vi "MFC Profile Generator.vi"(9 "Staircase Parameters":T1={"Step Time Duration"=1, "Step Flow Rate"=0.0, "Steps"=1, "Valve Open Start"=1, "Recovery"=FALSE, "Repeats"=1} {"Repeats" min=1 max=1000 step=1; "Valve Open Start" min=1 max=1000 step=1; "Steps" min=1 max=1000 step=1; "Step Flow Rate" min=0.0 max=200.0 scale=0.0..200.0; "Step Time Duration" min=1 max=1000 step=1}, 10 "Heaviside Step Parameters":T3 {"Valve Open Start" min=1 max=1000 step=1; "Valve Open Repeats" min=1 max=1000 step=1; "MFC Flow Rate" min=0.0 max=200.0 scale=0.0..200.0; "Valve Open Duration" min=1 max=1000 step=1}, 11 "Challenge Profile Type":T2) -> (3 "MFC Challenge Profile":dbl[](graph))   [LabVIEW 2011]
uses:
  Controls/MFC Challenge Profile - Heaviside Step.ctl
  Controls/MFC Challen Profile Type.ctl
  Controls/MFC Challenge Profile - Staircase.ctl
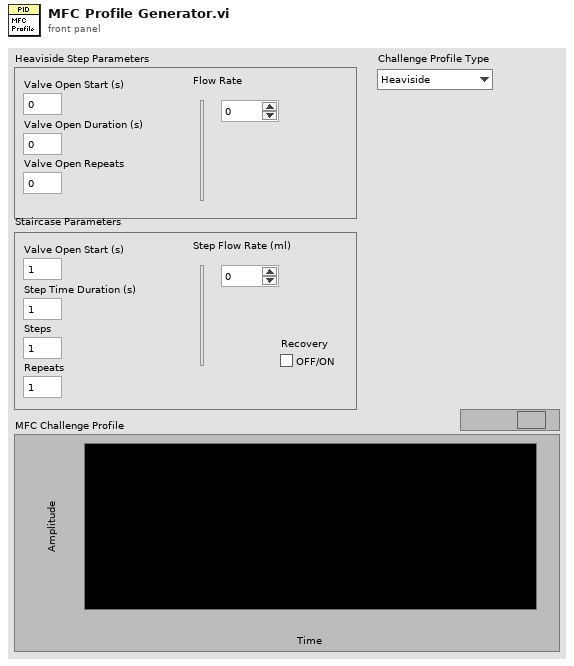
[diagram p1: front panel]
types:
  T1 = typedef "MFC Challenge Profile - Staircase.ctl" = cluster{"Step Time Duration":u16, "Step Flow Rate":dbl, "Steps":u16, "Valve Open Start":u16, "Recovery":bool, "Repeats":u16}
  T2 = typedef "MFC Challen Profile Type.ctl" = enum16{"Heaviside", "Staircase"}
  T3 = typedef "MFC Challenge Profile - Heaviside Step.ctl" = cluster{"Valve Open Duration":u16, "MFC Flow Rate":dbl, "Valve Open Repeats":u16, "Valve Open Start":u16}
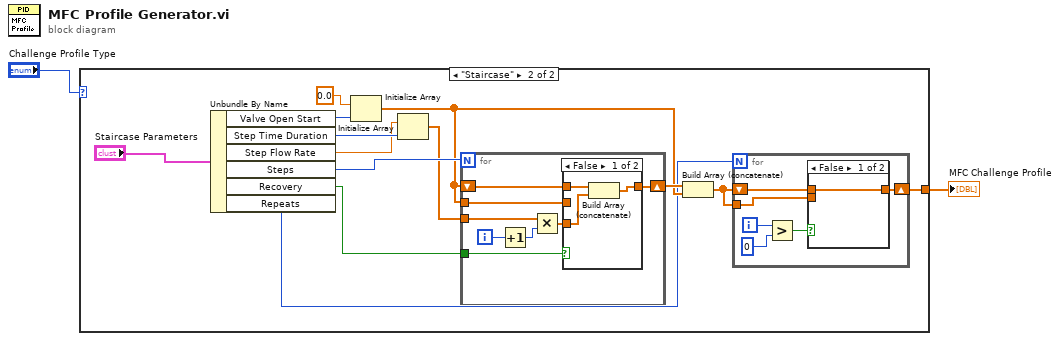
[diagram p0: block diagram]
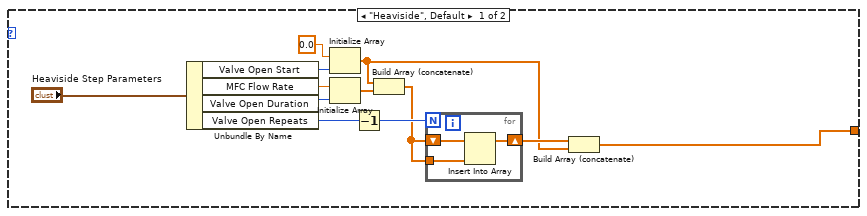
[diagram p2: hidden frame]
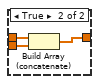
[diagram p3: hidden frame]
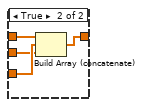
[diagram p4: hidden frame]
diagram:
  n1 = case shown="\"Staircase\"" "Challenge Profile Type" {
    tunnel: [w3 w18] -> w1
    frame "Heaviside", Default {
      n2 = Unbundle By Name("Heaviside Step Parameters") -> ("Valve Open Start"=w7:u16, "MFC Flow Rate"=w9:dbl, "Valve Open Duration"=w10:u16, "Valve Open Repeats"=w13:u16)
      n3 = Initialize Array(0.0 ("element"), w7) -> (w4:dbl[])
      n4 = Initialize Array(w9, w10) -> (w11:dbl[])
      n5 = Decrement(x=w13) -> (x-1=w14:u16)
      n6 = Build Array (concatenate)(w4, w11) -> (w12:dbl[])
      n7 = for {
        N: w14 -> [_]
        shift-right: [w15] -> w5
        shift-left: w12 -> [w17]
        tunnel: w12 -> [w16]
        n8 = Insert Into Array(array=w17, new element=w16) -> (w15:dbl[])  [unwired: 1 in]
      }
      n9 = Build Array (concatenate)(w5, w4) -> (w3:dbl[])
    }
    frame "Staircase" {
      n10 = Unbundle By Name("Staircase Parameters") -> ("Valve Open Start"=w28:u16, "Step Time Duration"=w27:u16, "Step Flow Rate"=w26:dbl, "Steps"=w25:u16, "Recovery"=w22:bool, "Repeats"=w19:u16)
      n11 = Initialize Array(0.0 ("element"), w28) -> (w21:dbl[])
      n12 = Initialize Array(w26, w27) -> (w24:dbl[])
      n13 = for {
        N: w25 -> [_]
        shift-right: [w45] -> w23
        shift-left: w21 -> [w47]
        tunnel: w24 -> [w48]
        tunnel: w22 -> [w42]
        tunnel: w21 -> [w41]
        i -> [w43]
        n14 = Increment(x=w43) -> (x+1=w44:i32)
        n15 = Multiply(x=w48, y=w44) -> (x*y=w46:dbl[])
        n16 = case shown="False" w42 {
          tunnel: w47 -> [w51 w55]
          tunnel: w46 -> [w50 w53]
          tunnel: [w49 w54] -> w45
          tunnel: w41 -> [_ w52]
          frame False {
            n17 = Build Array (concatenate)(w51, w50) -> (w49:dbl[])
          }
          frame True {
            n18 = Build Array (concatenate)(w55, w53, w52) -> (w54:dbl[])
          }
        }
      }
      n19 = Build Array (concatenate)(w23, w21) -> (w20:dbl[])
      n20 = for {
        N: w19 -> [_]
        shift-right: [w34] -> w18
        shift-left: w20 -> [w35]
        tunnel: w20 -> [w36]
        i -> [w33]
        n21 = Greater?(x=w33, y=0) -> (0:w31:bool)
        n22 = case shown="False" w31 {
          tunnel: w36 -> [_ w40]
          tunnel: w35 -> [w37 w39]
          tunnel: [w37 w38] -> w34
          frame False {
          }
          frame True {
            n23 = Build Array (concatenate)(w39, w40) -> (w38:dbl[])
          }
        }
      }
    }
  }
  "MFC Challenge Profile" <- w1
